vi "MLP_FS_Host.vi"() -> ()   [LabVIEW 2022 SP3]
uses:
  <vilib>/rvi/interface/nirviOpenFPGA/nirviOpenFPGA.xnode
  <vilib>/rvi/interface/nirviMethod/nirviMethod.xnode
  <vilib>/FPGAPlugInAG/Dynamic/niLvFpga_WriteFifo_Dynamic.vi
  <vilib>/rvi/errors/niLvFpgaMergeErrorWithErrorCode.vi
  <vilib>/FPGAPlugInAG/Dynamic/niLvFpga_Run_Dynamic.vi
  <vilib>/FPGAPlugInAG/Dynamic/niLvFpga_Reset_Dynamic.vi
  <vilib>/rvi/interface/nirviCloseFPGA/nirviCloseFPGA.xnode
  FPGA Bitfiles/mlpcontrollerfsp_FPGATarget_MLPFSTarget_Ulfa4tgwuzI.lvbitx
  MLP_FS_ Target.vi
  <vilib>/FPGAPlugInAG/cRIO-9054/niLvFpga_Open_cRIO-9054.vi
  <vilib>/rvi/interface/common/dynamic/niFpgaDynamicAddResources.vi
  <vilib>/FPGAPlugInAG/Dynamic/niLvFpga_ReadFifo_Dynamic.vi
  <vilib>/FPGAPlugInAG/Dynamic/niLvFpga_Close_Dynamic.vi
panel:
  out "Control Force":sgl[](graph)
  out "Uncontrolled Acceleration":dynamicdata(graph)
  out "Uncontrolled Velocity":dynamicdata(graph)
  out "Uncontrolled Displacement":dynamicdata(graph)
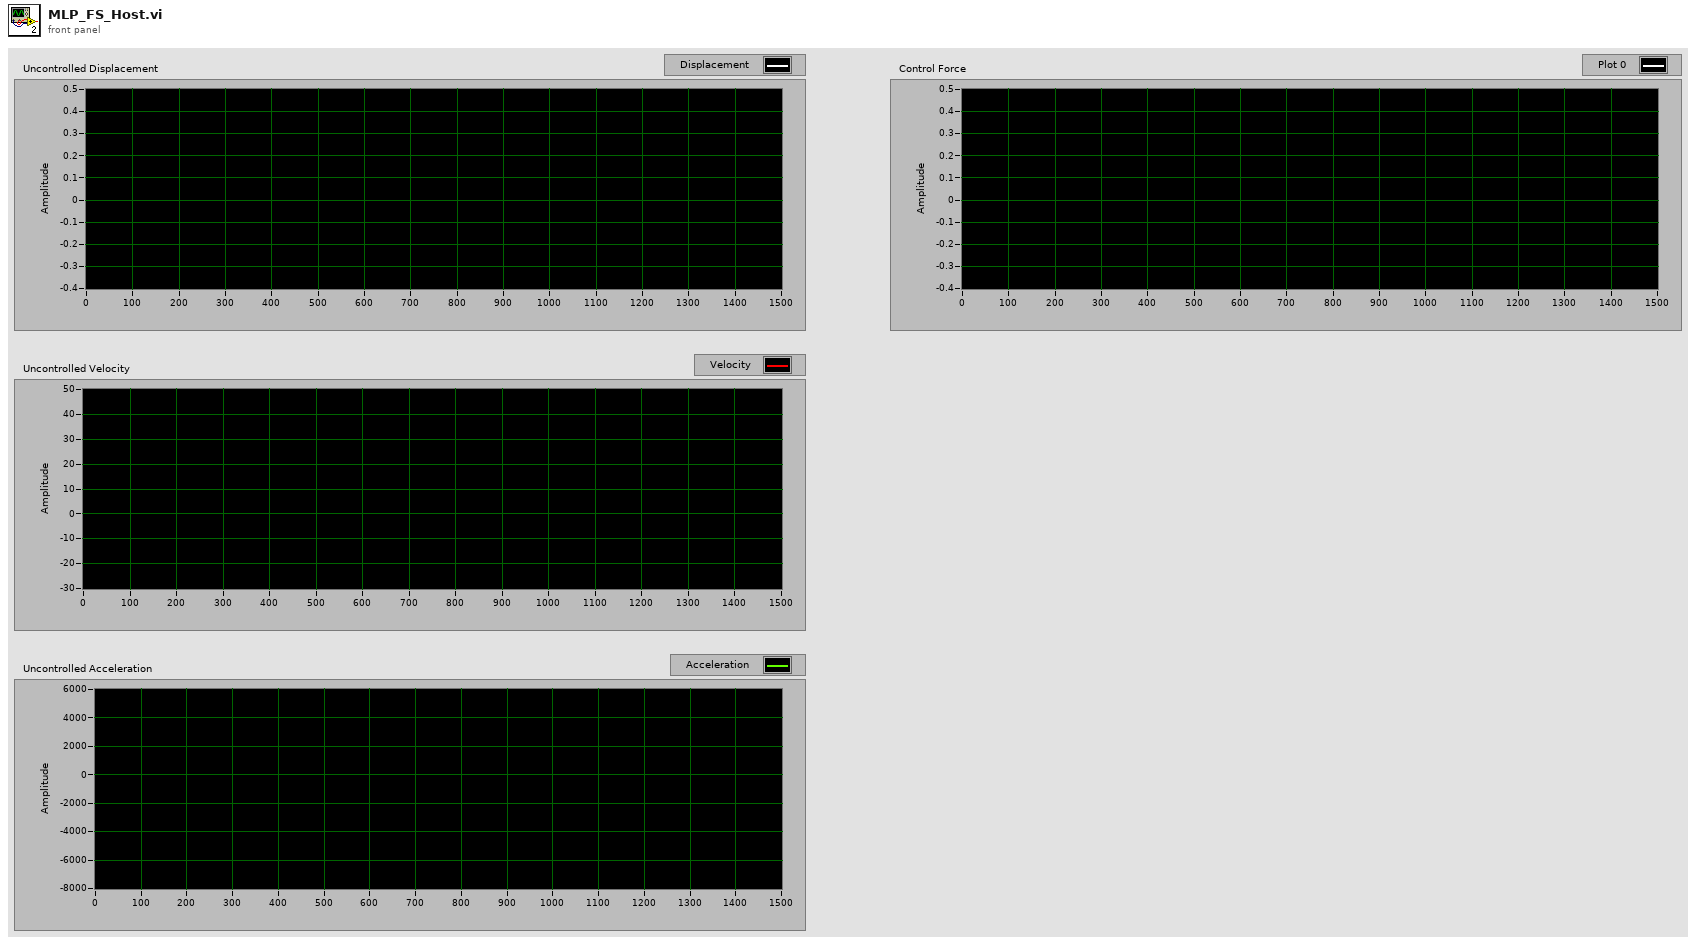
[diagram p1: front panel]
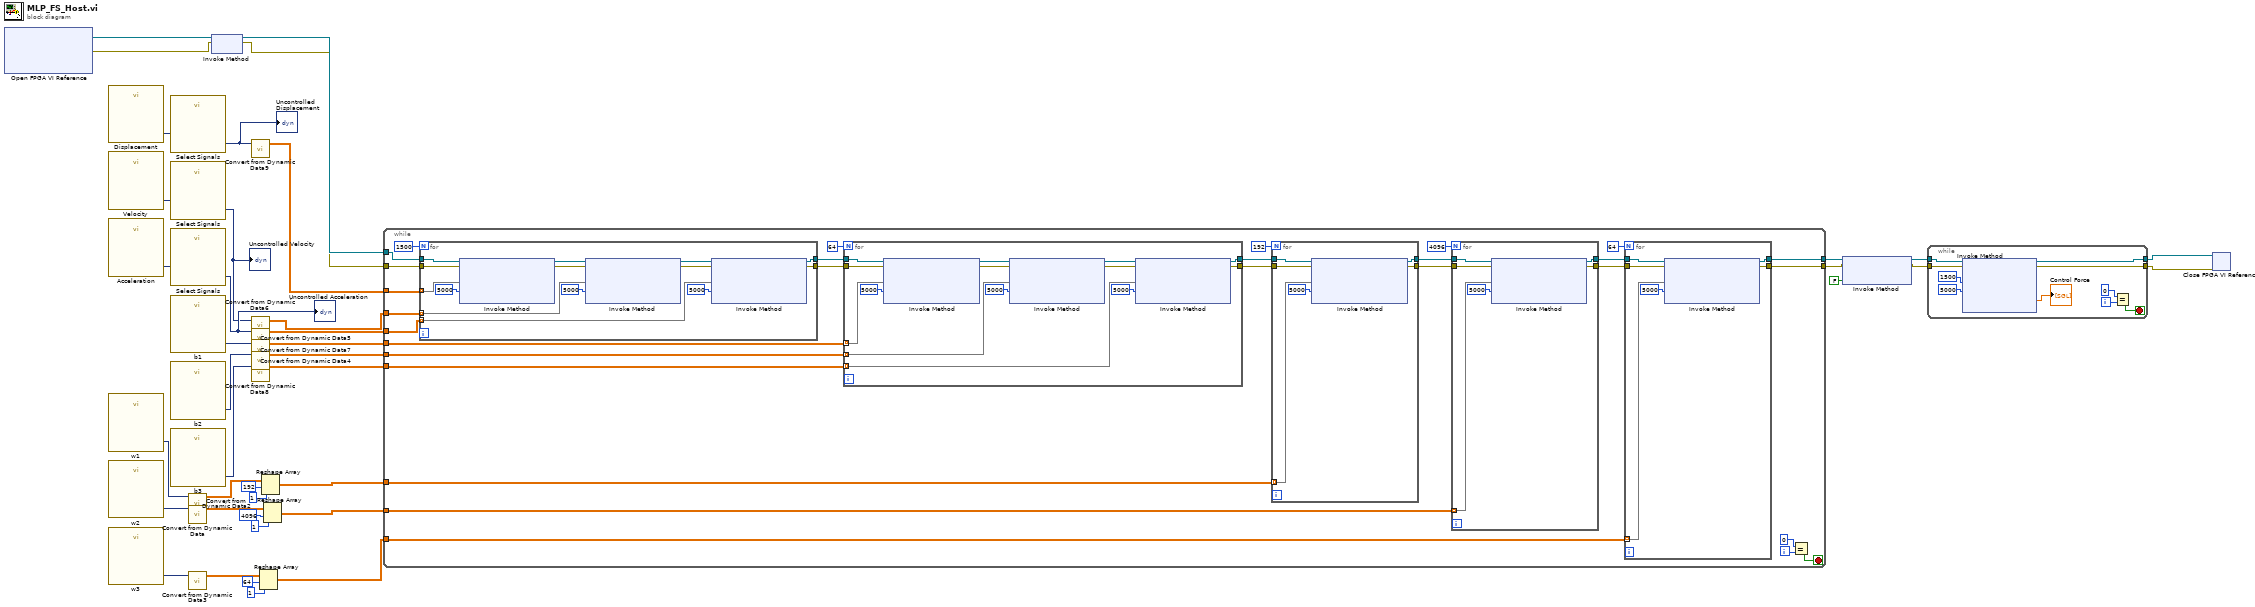
[diagram p0: block diagram]
diagram:
  n1 = xnode "Open FPGA VI Reference"() -> ("FPGA VI Reference Out"=w39:refnum<k20>, "error out"=w9:errorcluster)  [unwired: 2 in]
  n2 = call "Displacement"() -> ("Signals"=w23:dynamicdata)  [unwired: 6 in, 5 out]
  n3 = call "Velocity"() -> ("Signals"=w41:dynamicdata)  [unwired: 6 in, 5 out]
  n4 = call "Acceleration"() -> ("Signals"=w40:dynamicdata)  [unwired: 6 in, 5 out]
  n5 = call "w1"() -> ("Signals"=w34:dynamicdata)  [unwired: 6 in, 5 out]
  n6 = call "w2"() -> ("Signals"=w36:dynamicdata)  [unwired: 6 in, 5 out]
  n7 = call "w3"() -> ("Signals"=w30:dynamicdata)  [unwired: 6 in, 5 out]
  n8 = call "Select Signals"("Signals"=w23) -> ("Signal Out"=w3:dynamicdata)  [unwired: 9 in, 1 out]
  "Uncontrolled Displacement" <- w3
  n9 = call "Select Signals"("Signals"=w41) -> ("Signal Out"=w1:dynamicdata)  [unwired: 9 in, 1 out]
  "Uncontrolled Velocity" <- w1
  n10 = call "Select Signals"("Signals"=w40) -> ("Signal Out"=w2:dynamicdata)  [unwired: 9 in, 1 out]
  "Uncontrolled Acceleration" <- w2
  n11 = call "b1"() -> ("Signals"=w29:dynamicdata)  [unwired: 6 in, 5 out]
  n12 = call "b2"() -> ("Signals"=w28:dynamicdata)  [unwired: 6 in, 5 out]
  n13 = call "b3"() -> ("Signals"=w27:dynamicdata)  [unwired: 6 in, 5 out]
  n14 = call "Convert from Dynamic Data2"("Dynamic Data Type"=w34) -> ("Array"=w33:dbl[][])  [unwired: 3 in]
  n15 = call "Convert from Dynamic Data"("Dynamic Data Type"=w36) -> ("Array"=w35:dbl[][])  [unwired: 3 in]
  n16 = call "Convert from Dynamic Data3"("Dynamic Data Type"=w30) -> ("Array"=w31:dbl[][])  [unwired: 3 in]
  n17 = xnode "Invoke Method"("FPGA VI Reference In"=w39, "error in"=w9) -> ("FPGA VI Reference Out"=w11:refnum<k20>, "error out"=w10:errorcluster)
  n18 = call "Convert from Dynamic Data9"("Dynamic Data Type"=w3) -> ("Array"=w14:dbl[][])  [unwired: 3 in]
  n19 = call "Convert from Dynamic Data6"("Dynamic Data Type"=w1) -> ("Array"=w12:dbl[][])  [unwired: 3 in]
  n20 = call "Convert from Dynamic Data5"("Dynamic Data Type"=w2) -> ("Array"=w13:dbl[][])  [unwired: 3 in]
  n21 = call "Convert from Dynamic Data7"("Dynamic Data Type"=w29) -> ("Array"=w15:dbl[][])  [unwired: 3 in]
  n22 = call "Convert from Dynamic Data4"("Dynamic Data Type"=w28) -> ("Array"=w17:dbl[][])  [unwired: 3 in]
  n23 = call "Convert from Dynamic Data8"("Dynamic Data Type"=w27) -> ("Array"=w16:dbl[][])  [unwired: 3 in]
  n24 = Reshape Array(w31, 64 ("dimension size"), 1 ("dimension size")) -> (w24:dbl[][])
  n25 = Reshape Array(w33, 192 ("dimension size"), 1 ("dimension size")) -> (w26:dbl[][])
  n26 = Reshape Array(w35, 4096 ("dimension size"), 1 ("dimension size")) -> (w25:dbl[][])
  n27 = while {
    tunnel: w11 -> [w70]
    tunnel: w10 -> [w68]
    tunnel: w12 -> [w55]
    tunnel: w13 -> [w54]
    tunnel: w15 -> [w53]
    tunnel: w17 -> [w52]
    tunnel: w26 -> [w42]
    tunnel: w25 -> [w43]
    tunnel: w24 -> [w44]
    tunnel: [w51] -> w21
    tunnel: [w50] -> w20
    tunnel: w16 -> [w46]
    tunnel: w14 -> [w45]
    i -> [w49]
    stop <- w47 stop-if-true
    n28 = for {
      N: 1500 -> [_]
      tunnel: w70 -> [w116]
      tunnel: w68 -> [w113]
      tunnel: [w110] -> w63
      tunnel: [w109] -> w62
      tunnel: w55 -> [w104] mode=indexing
      tunnel: w54 -> [w103] mode=indexing
      tunnel: w45 -> [w105] mode=indexing
      n29 = xnode "Invoke Method"("FPGA VI Reference In"=w116, "error in"=w113, "Data"=w105, "Timeout (ms)"=5000) -> ("FPGA VI Reference Out"=w115:refnum<k20>, "error out"=w114:errorcluster)  [unwired: 1 out]
      n30 = xnode "Invoke Method"("FPGA VI Reference In"=w115, "error in"=w114, "Data"=w104, "Timeout (ms)"=5000) -> ("FPGA VI Reference Out"=w111:refnum<k20>, "error out"=w112:errorcluster)  [unwired: 1 out]
      n31 = xnode "Invoke Method"("FPGA VI Reference In"=w111, "error in"=w112, "Data"=w103, "Timeout (ms)"=5000) -> ("FPGA VI Reference Out"=w110:refnum<k20>, "error out"=w109:errorcluster)  [unwired: 1 out]
    }
    n32 = for {
      N: 64 -> [_]
      tunnel: w63 -> [w98]
      tunnel: w62 -> [w97]
      tunnel: [w96] -> w61
      tunnel: [w95] -> w60
      tunnel: w53 -> [w89] mode=indexing
      tunnel: w52 -> [w91] mode=indexing
      tunnel: w46 -> [w90] mode=indexing
      n33 = xnode "Invoke Method"("FPGA VI Reference In"=w98, "error in"=w97, "Data"=w89, "Timeout (ms)"=5000) -> ("FPGA VI Reference Out"=w102:refnum<k20>, "error out"=w101:errorcluster)  [unwired: 1 out]
      n34 = xnode "Invoke Method"("FPGA VI Reference In"=w102, "error in"=w101, "Data"=w91, "Timeout (ms)"=5000) -> ("FPGA VI Reference Out"=w99:refnum<k20>, "error out"=w100:errorcluster)  [unwired: 1 out]
      n35 = xnode "Invoke Method"("FPGA VI Reference In"=w99, "error in"=w100, "Data"=w90, "Timeout (ms)"=5000) -> ("FPGA VI Reference Out"=w96:refnum<k20>, "error out"=w95:errorcluster)  [unwired: 1 out]
    }
    n36 = for {
      N: 192 -> [_]
      tunnel: w61 -> [w88]
      tunnel: w60 -> [w87]
      tunnel: [w86] -> w59
      tunnel: [w85] -> w58
      tunnel: w42 -> [w84] mode=indexing
      n37 = xnode "Invoke Method"("FPGA VI Reference In"=w88, "error in"=w87, "Data"=w84, "Timeout (ms)"=5000) -> ("FPGA VI Reference Out"=w86:refnum<k20>, "error out"=w85:errorcluster)  [unwired: 1 out]
    }
    n38 = for {
      N: 4096 -> [_]
      tunnel: w59 -> [w82]
      tunnel: w58 -> [w81]
      tunnel: [w80] -> w57
      tunnel: [w79] -> w56
      tunnel: w43 -> [w78] mode=indexing
      n39 = xnode "Invoke Method"("FPGA VI Reference In"=w82, "error in"=w81, "Data"=w78, "Timeout (ms)"=5000) -> ("FPGA VI Reference Out"=w80:refnum<k20>, "error out"=w79:errorcluster)  [unwired: 1 out]
    }
    n40 = for {
      N: 64 -> [_]
      tunnel: w57 -> [w76]
      tunnel: w56 -> [w75]
      tunnel: w44 -> [w71] mode=indexing
      tunnel: [w73] -> w51
      tunnel: [w72] -> w50
      n41 = xnode "Invoke Method"("FPGA VI Reference In"=w76, "error in"=w75, "Data"=w71, "Timeout (ms)"=5000) -> ("FPGA VI Reference Out"=w73:refnum<k20>, "error out"=w72:errorcluster)  [unwired: 1 out]
    }
    n42 = Equal?(x=0, y=w49) -> (x = y?=w47:bool)
  }
  n43 = xnode "Invoke Method"("FPGA VI Reference In"=w21, "error in"=w20, "Wait Until Done (F)"=FALSE) -> ("FPGA VI Reference Out"=w19:refnum<k20>, "error out"=w18:errorcluster)
  n44 = while {
    tunnel: w19 -> [w126]
    tunnel: [w121] -> w5
    tunnel: w18 -> [w123]
    tunnel: [w122] -> w4
    i -> [w118]
    stop <- w119 stop-if-true
    n45 = xnode "Invoke Method"("FPGA VI Reference In"=w126, "error in"=w123, "Number of Elements"=u32 1500, "Timeout (ms)"=5000) -> ("FPGA VI Reference Out"=w121:refnum<k20>, "error out"=w122:errorcluster, "Data"=→"Control Force":sgl[])  [unwired: 1 out]
    n46 = Equal?(x=0, y=w118) -> (x = y?=w119:bool)
  }
  n47 = xnode "Close FPGA VI Reference"("FPGA VI Reference In"=w5, "error in"=w4) -> ()  [unwired: 1 out]
